vi "as_genStimList.vi"(10 "Stimulus Parameters":dbl[][](array[numeric])=[[3.0, 200.0, 1.0, 500.0], [3.0, 200.0, 1.0, 1000.0]], 11 "Repetitions":i32=10 caption="# of Random Repetitions for Each Stimulus" min=2) -> (2 "Stimulus List":dbl[][](array[numeric]))   [LabVIEW 2013]
panel:
  # "Stim#, Stim Type, Duration, Amplitude, Param 1, Param 2, Param 3, Param 4"
  # "Stim Type, Duration, Amplitude, Param 1, Param 2, Param 3, Param 4"
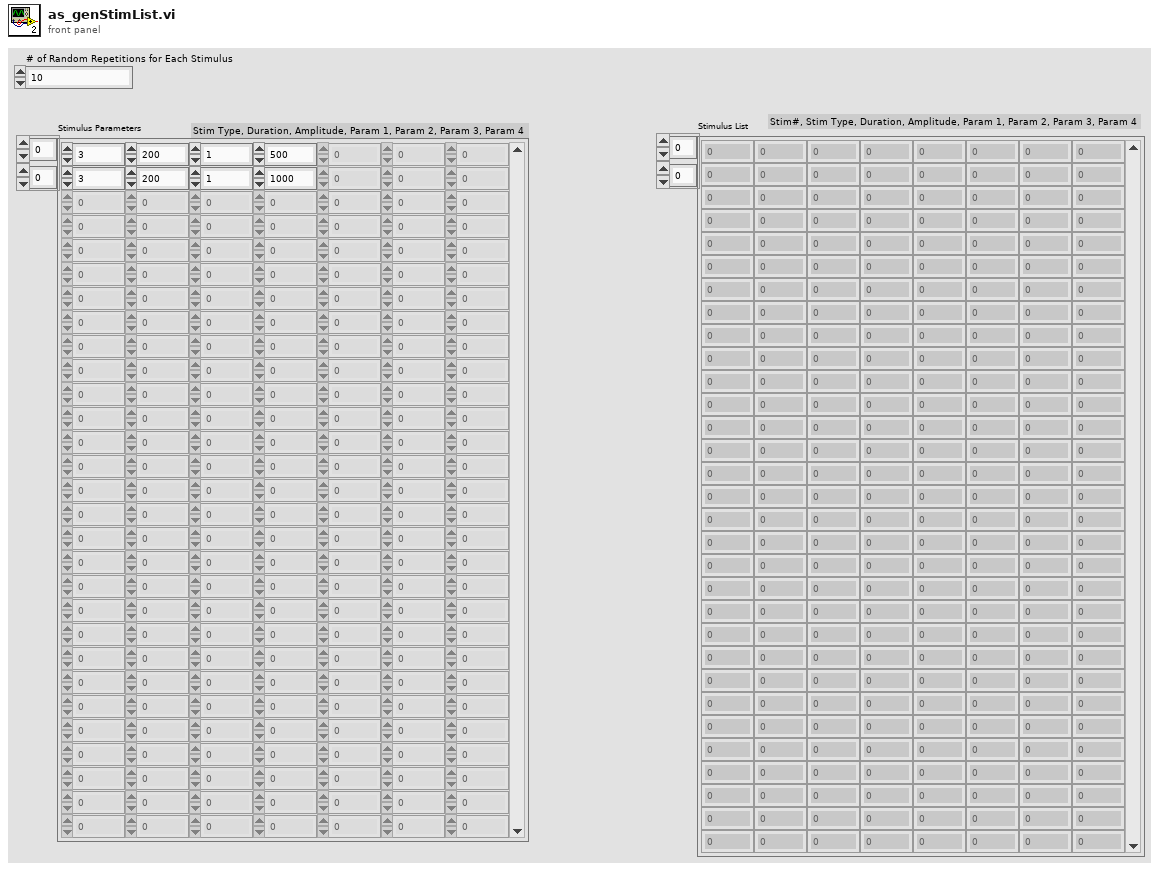
[diagram p1: front panel]
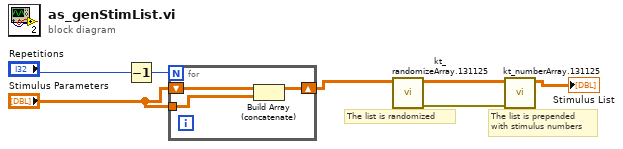
[diagram p0: block diagram]
diagram:
  # "The list is prepended\nwith stimulus numbers"
  # "The list is randomized"
  n1 = Decrement(x="Repetitions") -> (x-1=w7:i32)
  n2 = for {
    N: w7 -> [_]
    shift-right: [w10] -> w6
    shift-left: "Stimulus Parameters" -> [w9]
    tunnel: "Stimulus Parameters" -> [w8]
    n3 = Build Array (concatenate)(w9, w8) -> (w10:dbl[][])
  }
  n4 = call "kt_randomizeArray.131125.vi"("Array In"=w6) -> ("error out"=w4:errorcluster, "Array Out"=w5:dbl[][])  [unwired: 9 in]
  n5 = call "kt_numberArray.131125.vi"("error in (no error)"=w4, "Array In"=w5) -> ("Array Out"=→"Stimulus List":dbl[][])  [unwired: 8 in, 1 out]
